vi "old_Ballard - 1553 RT Driver VI.vi"(7 "Operation":T1, 11 "Device Reference in":T2 format="%.0x") -> (0 "Error Code":i32)   [LabVIEW 2017]
uses:
  <vilib>/NI Veristand/Custom Device API/Custom Device Item Ref.ctl
  <vilib>/NI Veristand/Custom Device API/Hardware Interface Driver VI Operation.ctl
  RT Driver/Controls/RT StateVariables.ctl
  <vilib>/NI/NIVS Inline Async API/_VS Inline Async API/VS Inline Async API/VS Inline Async API.lvclass
  RT Driver/Controls/Card Parameters.ctl
  Shared/Controls and Global/Initialization Method.ctl
  <vilib>/NI Veristand/Custom Device API/Data Reference.ctl
  RT Driver/Controls/RT Inline Data_Data Description_Channel.ctl
  RT Driver/Controls/RT Inline Frame Descriptor.ctl
  RT Driver/Controls/RT Inline Frame Descriptor_BC.ctl
  <vilib>/NI Veristand/Custom Device API/Block Data Reference.ctl
  RT Driver/Controls/RT Inline Frame Descriptor_RT.ctl
  Shared/Controls and Global/RT CWD2.ctl
  Shared/Controls and Global/RT CWD1.ctl
  Shared/Controls and Global/RT messageType.ctl
  RT Driver/Controls/Inline_Status_Channels.ctl
  <vilib>/NI Veristand/Custom Device API/Custom Device API.lvlib
  <vilib>/NI VeriStand/Custom Device Tools/Custom Device Utility Library/Custom Device Utility Library.lvlib
  Ballard MIL-1553 Engine.lvlib
  Shared/Ballard 1553 Shared.lvlib
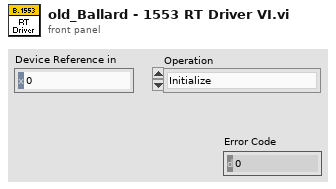
[diagram p1: front panel]
types:
  T1 = typedef "Custom Device API.lvlib/Hardware Interface Driver VI Operation.ctl" = enum16{"Initialize", "Start", "Read Data from HW", "Write Data to HW", "Close"}
  T2 = typedef "Custom Device API.lvlib/Custom Device Item Ref.ctl" = u64
  T3 = typedef "Ballard MIL-1553 Engine.lvlib/RT StateVariables.ctl" = cluster{"Async":refnum<class "VS Inline Async API.lvclass">, "Card Parameters (out)":T4, "Inline Status Channels Refs":T6[], "RT Inline Data_Data Description_Channels":T7[]}
  T4 = typedef "Ballard MIL-1553 Engine.lvlib/Card Parameters.ctl" = cluster{"card number":i32, "core number":i32, "core handle":u64, "core reader handle":u64, "channel handles[]":u64[], "Initialization Method":T5, "PXI slot number":i32}
  T5 = typedef "Ballard 1553 Shared.lvlib/Initialization Method.ctl" = enum16{"PXI Slot Number", "Card Number"}
  T6 = typedef "Custom Device API.lvlib/Data Reference.ctl" = i32
  T7 = typedef "Ballard MIL-1553 Engine.lvlib/RT Inline Data_Data Description_Channel.ctl" = cluster{"hardwareChannel":u16, "First Index for RT2RT Frames":i32, "Frame Drescriptors":T8[]}
  T8 = typedef "Ballard MIL-1553 Engine.lvlib/RT Inline Frame Descriptor.ctl" = cluster{"BC":T9, "RT":T11, "Initialized?":bool, "RT to RT?":bool, "CWD2":T12, "CWD1":T13, "messageType":T14, "Name":string}
  T9 = typedef "Ballard MIL-1553 Engine.lvlib/RT Inline Frame Descriptor_BC.ctl" = cluster{"Timestamp?":bool, "Timestamp Channel Ref":T2, "Data Words?":bool, "Words Block Data Refs":T10[], "Sw1?":bool, "Sw2?":bool, "Status Channel Refs":T2[]}
  T10 = typedef "Custom Device API.lvlib/Block Data Reference.ctl" = cluster{"Data Reference":T6, "Offset":u64, "Length":u64}
  T11 = typedef "Ballard MIL-1553 Engine.lvlib/RT Inline Frame Descriptor_RT.ctl" = cluster{"Timestamp?":bool, "Timestamp Channel Ref":T2, "Data Words?":bool, "Words Block Data Refs":T10[], "Status Channel Ref?":bool, "Status Channel Ref":T2}
  T12 = typedef "Ballard 1553 Shared.lvlib/RT CWD2.ctl" = cluster{"TA (RT)":i8, "SA":i8, "Words (WC)":i8}
  T13 = typedef "Ballard 1553 Shared.lvlib/RT CWD1.ctl" = cluster{"TA (RT)":i8, "SA":i8, "Mode Code":i8, "Words Count":i8}
  T14 = typedef "Ballard 1553 Shared.lvlib/RT messageType.ctl" = enum16{"BC to RT", "RT to BC", "RT to RT", "MC (Rx)", "MC (Tx)"}
  T15 = typedef "Ballard MIL-1553 Engine.lvlib/Inline_Status_Channels.ctl" = enum16{"Error Code", "Inline Read Time (us)", "Inline Write Time (us)", "Unconfigured Frames Counter", "Monitor - Error Counter", "General Protocol Error Counter", "Wrong Sync Error Counter", "Improper Number of Data Words Error", "Manchester Error Counter", "Parity Error Counter", "Word Error Counter"}
  T16 = typedef "Ballard MIL-1553 Engine.lvlib/RT Async Data.ctl" = cluster{"Map (BC to RT)":T17[], "Raw Values (BC to RT)":T19, "Map (RT to ..)":T21[], "Raw Values (RT to ..)":T19, "Map (RTs Status)":T22[], "Raw Values (RTs Status)":T19, "Map (Bc Command Channels)":T23[], "MAP (BC Acyclic Messages Trigger)":T24[], "Map (RT Command Channels)":T25[], "Map (MC Rx)":T26[]}
  T17 = typedef "Ballard MIL-1553 Engine.lvlib/RT Async_Map BC2RT.ctl" = cluster{"Channel Index":i32, "ID":i32, "Channel Data Reference":T6, "Word Index":i32, "Message Handle":u64, "Type":T18}
  T18 = typedef "Ballard MIL-1553 Engine.lvlib/RT Async_Map_Type.ctl" = enum16{"Word (BC to RT)", "Word (MC (Rx))", "Acyclic Message Trigger", "Word (RT to ..)", "Word (RT to RT)", "Word (MC (Tx))", "RT Status", "BC Commands", "RT Commands"}
  T19 = typedef "Ballard MIL-1553 Engine.lvlib/RT Async_Raw Values.ctl" = cluster{"Association":T20[], "Raw Values Array":u16[]}
  T20 = typedef "Ballard MIL-1553 Engine.lvlib/RT Async_Raw Values_Association.ctl" = cluster{"Channel Data Reference":T6, "Raw Value Index":i32}
  T21 = typedef "Ballard MIL-1553 Engine.lvlib/RT Async_Map RT2BC.ctl" = cluster{"Channel Index":i32, "ID":i32, "Word Data Reference":T6, "Word Index":i32, "rt Transfer Handle":u64, "Type":T18}
  T22 = typedef "Ballard MIL-1553 Engine.lvlib/RT Async_Map RTs Status.ctl" = cluster{"Channel Index":i32, "ID":i32, "rt Transfer Handle":u64, "Type":T18}
  T23 = typedef "Ballard MIL-1553 Engine.lvlib/RT Async_Map BC Command Channels.ctl" = cluster{"Channel Index":i32, "ID":i32, "BC Handle":u64, "Type":T18, "BC Command Channel Ref":T2, "Command Type":enum16{"Start Command", "Stop Command"}}
  T24 = typedef "Ballard MIL-1553 Engine.lvlib/RT Async_Map BC Acyclic Messages Trigger.ctl" = cluster{"Channel Index":i32, "BC Handle":u64, "Type":T18, "Acyclic Message Trigger Channel Ref":T2, "Message Name":string}
  T25 = typedef "Ballard MIL-1553 Engine.lvlib/RT Async_Map RT Command Channels.ctl" = cluster{"Channel Index":i32, "ID":i32, "RT Handle":u64, "Type":T18, "RT Command Channel Ref":T2, "Command Type":enum16{"Start Command", "Stop Command"}}
  T26 = typedef "Ballard MIL-1553 Engine.lvlib/RT Async_Map MC Rx.ctl" = cluster{"Channel Index":i32, "ID":i32, "Channel Data Reference":T6, "Word Index":i32, "Message Handle":u64, "Type":T18}
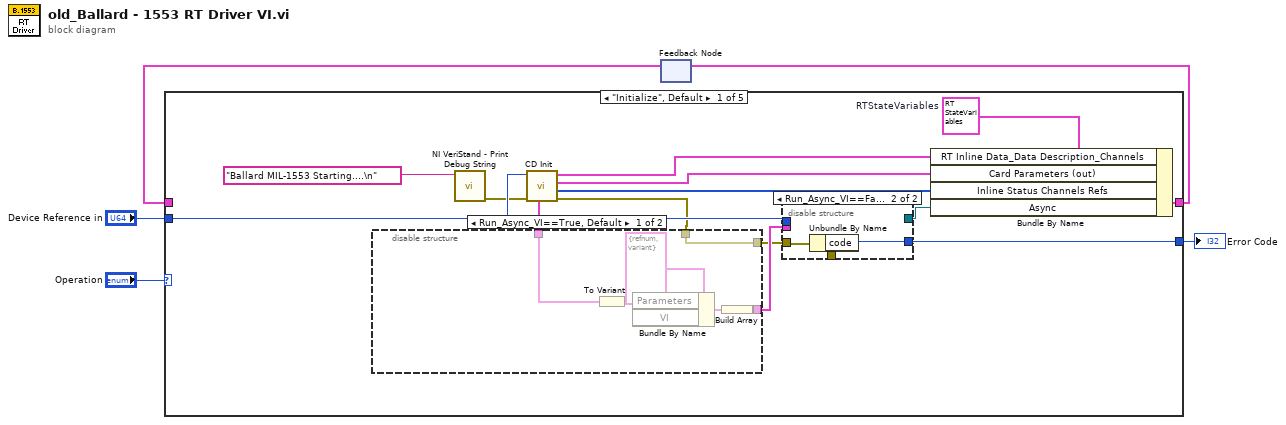
[diagram p0: block diagram]
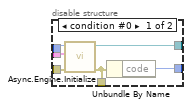
[diagram p3: hidden frame]
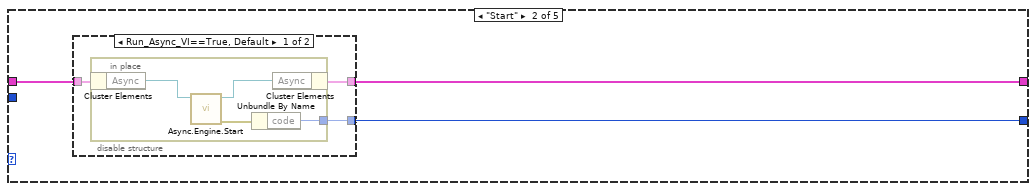
[diagram p4: hidden frame]
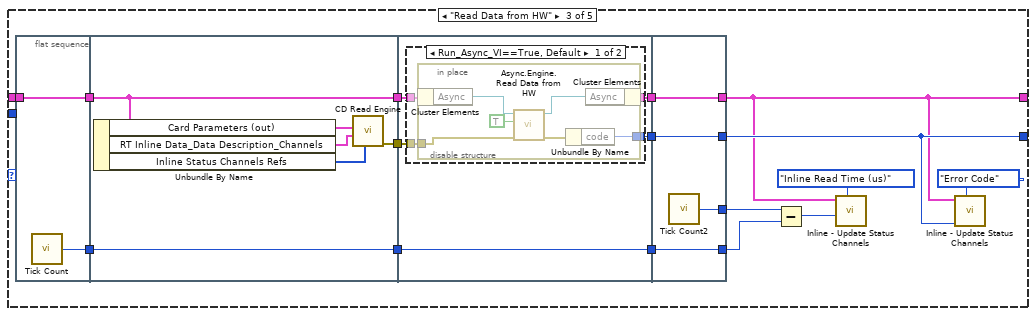
[diagram p6: hidden frame]
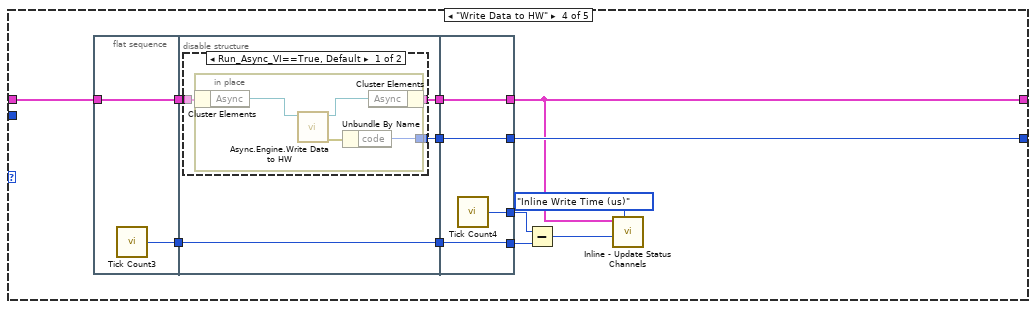
[diagram p8: hidden frame]
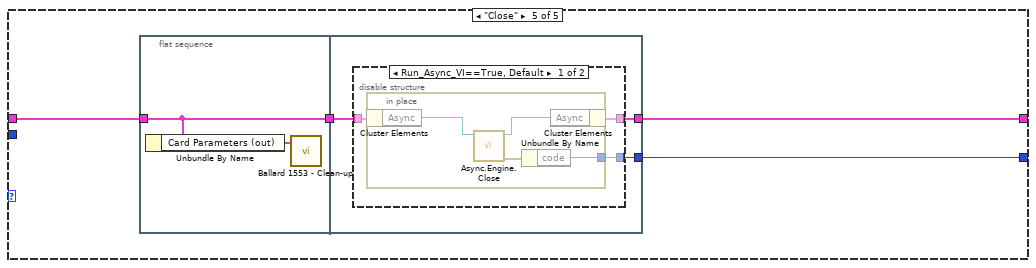
[diagram p10: hidden frame]
diagram:
  n1 = feedback #1() -> (w3:T3)  [unwired: 1 out]
  n2 = case shown="\"Initialize\", Default" "Operation" {
    tunnel: [w17 w36 w53 w91 w122] -> w4
    tunnel: w3 -> [_ w37 w61 w100 w123]
    tunnel: "Device Reference in" -> [w13 _ _ _ _]
    tunnel: [w19 w35 w56 w101 w121] -> w1
    frame "Initialize", Default {
      w16 = T3 {"Async"=refnum, "Card Parameters (out)"={"card number"=0, "core number"=0, "core handle"=0, "core reader handle"=0, "channel handles[]"=[], "Initialization Method"=enum."PXI Slot Number", "PXI slot number"=0}, "Inline Status Channels Refs"=[], "RT Inline Data_Data Description_Channels"=[]}  # RTStateVariables
      n3 = call <vilib>:"NI VeriStand - Print Debug String.vi"("Message"="Ballard MIL-1553 Starting....\n") -> ("error out"=w9:errorcluster)  [unwired: 10 in]
      n4 = call "CD Init.vi"("Error (in)"=w9, "Device Reference"=w13) -> ("Error (out)"=w7:errorcluster, "Inline Status Channels Refs"=w10:T6[], "Card Parameters (out)"=w11:T4, "RT Inline Data_Data Description_Channels"=w12:T7[], "RT Async Data"=w8:T16)  [unwired: 5 in]
      n5 = disable-structure shown="Run_Async_VI==True, Default" {
        disable-tunnel: [w23 _] -> w15
        disable-tunnel: w8 -> [w21 _]
        disable-tunnel: w7 -> [w20 w26]
        disable-tunnel: [w20 w26] -> w6
        frame condition #0 {
          n6 = To Variant(anything=w21) -> (Variant=w22:variant)
          n7 = Bundle By Name(cluster=cluster{"VI":refnum<vi>, "Parameters":variant} {"VI"=refnum, "Parameters"=variant} ("Process"), "Parameters"=w22) -> (w24:cluster{"VI":refnum<vi>, "Parameters":variant})  [unwired: 1 in]
          n8 = Build Array(w24) -> (w23:cluster{"VI":refnum<vi>, "Parameters":variant}[])
        }
        frame condition #1 (active) {
        }
      }
      n9 = disable-structure shown="Run_Async_VI==False" {
        disable-tunnel: [w32 w33] -> w19
        disable-tunnel: [w31 _] -> w18
        disable-tunnel: w15 -> [w30 _]
        disable-tunnel: w6 -> [w29 w34]
        disable-tunnel: w13 -> [w28 _]
        disable-tunnel: [w27 _] -> _
        frame condition #0 {
          n10 = call <vilib>:"Async.Engine.Initialize.vi"("error in (no error)"=w29, "Processes"=w30, "Custom Device Ref"=w28) -> ("error out"=w27:errorcluster, "Async"=w31:refnum<class "VS Inline Async API.lvclass">)  [unwired: 7 in]
          n11 = Unbundle By Name(w27) -> ("code"=w32:i32)
        }
        frame condition #1 (active) {
          n12 = Unbundle By Name(w34) -> ("code"=w33:i32)
        }
      }
      n13 = Bundle By Name(cluster=w16, "RT Inline Data_Data Description_Channels"=w12, "Card Parameters (out)"=w11, "Inline Status Channels Refs"=w10, "Async"=w18) -> (w17:T3)
    }
    frame "Start" {
      n14 = disable-structure shown="Run_Async_VI==True, Default" {
        disable-tunnel: w37 -> [w40 w45]
        disable-tunnel: [w39 w45] -> w36
        disable-tunnel: [w38 _] -> w35
        frame condition #0 {
          n15 = in-place {
            in-place-border: [w41] -> w38
            n16 = in-place-cluster #2(w40) -> ("Async"=w44:refnum<class "VS Inline Async API.lvclass">)
            n17 = call <vilib>:"Async.Engine.Start.vi"("VS Inline Async API in"=w44) -> ("error out"=w42:errorcluster, "VS Inline Async API out"=w43:refnum<class "VS Inline Async API.lvclass">)  [unwired: 9 in]
            n18 = Unbundle By Name(w42) -> ("code"=w41:i32)
            n19 = in-place-cluster #2("Async"=w43) -> (w39:T3)
          }
        }
        frame condition #1 (active) {
        }
      }
    }
    frame "Read Data from HW" {
      n20 = flat-sequence {
        tunnel: w61 -> [w63]
        tunnel: [w63] -> w60
        tunnel: [w62] -> w59
        tunnel: [w68] -> w52
        tunnel: [w69] -> w50
        tunnel: w59 -> [w69]
        tunnel: w60 -> [w68]
        tunnel: [w67] -> w47
        tunnel: w52 -> [w72]
        tunnel: [w71] -> w51
        tunnel: w50 -> [w74]
        tunnel: [w74] -> w49
        tunnel: [w73] -> w48
        tunnel: w47 -> [w70]
        tunnel: [w88] -> w53
        tunnel: [w89] -> w56
        tunnel: w51 -> [w88]
        tunnel: [w87] -> w58
        tunnel: w49 -> [w86]
        tunnel: [w86] -> w57
        tunnel: w48 -> [w89]
        frame #0 {
          n21 = call "Tick Count"() -> ("Tick Count(uSec)"=w62:u32)
        }
        frame #1 {
          n22 = Unbundle By Name(w68) -> ("Card Parameters (out)"=w66:T4, "RT Inline Data_Data Description_Channels"=w64:T7[], "Inline Status Channels Refs"=w65:T6[])
          n23 = call "CD Read Engine.vi"("Inline Status Channels Refs"=w65, "RT Inline Data_Data Description_Channels"=w64, "Card Parameters (in)"=w66) -> ("Error (out)"=w67:errorcluster)  [unwired: 7 in]
        }
        frame #2 {
          n24 = disable-structure shown="Run_Async_VI==True, Default" {
            disable-tunnel: [w78 _] -> w73
            disable-tunnel: w72 -> [w77 w85]
            disable-tunnel: [w76 w85] -> w71
            disable-tunnel: w70 -> [w75 _]
            frame condition #0 {
              n25 = in-place {
                in-place-border: [w82] -> w78
                in-place-border: w75 -> [w79]
                n26 = in-place-cluster #3(w77) -> ("Async"=w84:refnum<class "VS Inline Async API.lvclass">)
                n27 = call <vilib>:"Async.Engine.Read Data from HW.vi"("error in"=w79, "Report Error to Inline?"=TRUE, "Async in"=w84) -> ("error out"=w81:errorcluster, "Async out"=w83:refnum<class "VS Inline Async API.lvclass">)  [unwired: 7 in]
                n28 = Unbundle By Name(w81) -> ("code"=w82:i32)
                n29 = in-place-cluster #3("Async"=w83) -> (w76:T3)
              }
            }
            frame condition #1 (active) {
            }
          }
        }
        frame #3 {
          n30 = call "Tick Count2"() -> ("Tick Count(uSec)"=w87:u32)
        }
      }
      n31 = Subtract(x=w58, y=w57) -> (x-y=w54:u32)
      n32 = call "Inline - Update Status Channels.vi"("Status Channel"=Inline_Status_Channels."Inline Read Time (us)", "Time (us)"=w54, "RTStateVariables"=w53) -> ()  [unwired: 9 in]
      n33 = call "Inline - Update Status Channels.vi"("Status Channel"=Inline_Status_Channels."Error Code", "Error Code"=w56, "RTStateVariables"=w53) -> ()  [unwired: 9 in]
    }
    frame "Write Data to HW" {
      n34 = flat-sequence {
        tunnel: w100 -> [w103]
        tunnel: [w103] -> w99
        tunnel: [w102] -> w96
        tunnel: w99 -> [w104]
        tunnel: [w107] -> w98
        tunnel: [w106] -> w97
        tunnel: w96 -> [w105]
        tunnel: [w105] -> w95
        tunnel: [w118] -> w91
        tunnel: [w119] -> w101
        tunnel: w98 -> [w119]
        tunnel: w97 -> [w118]
        tunnel: [w117] -> w93
        tunnel: w95 -> [w116]
        tunnel: [w116] -> w94
        frame #0 {
          n35 = call "Tick Count3"() -> ("Tick Count(uSec)"=w102:u32)
        }
        frame #1 {
          n36 = disable-structure shown="Run_Async_VI==True, Default" {
            disable-tunnel: [w110 _] -> w107
            disable-tunnel: w104 -> [w109 w115]
            disable-tunnel: [w108 w115] -> w106
            frame condition #0 {
              n37 = in-place {
                in-place-border: [w114] -> w110
                n38 = in-place-cluster #4(w109) -> ("Async"=w112:refnum<class "VS Inline Async API.lvclass">)
                n39 = call <vilib>:"Async.Engine.Write Data to HW.vi"("VS Inline Async API in"=w112) -> ("error out"=w113:errorcluster, "VS Inline Async API out"=w111:refnum<class "VS Inline Async API.lvclass">)  [unwired: 9 in]
                n40 = Unbundle By Name(w113) -> ("code"=w114:i32)
                n41 = in-place-cluster #4("Async"=w111) -> (w108:T3)
              }
            }
            frame condition #1 (active) {
            }
          }
        }
        frame #2 {
          n42 = call "Tick Count4"() -> ("Tick Count(uSec)"=w117:u32)
        }
      }
      n43 = Subtract(x=w93, y=w94) -> (x-y=w92:u32)
      n44 = call "Inline - Update Status Channels.vi"("Status Channel"=Inline_Status_Channels."Inline Write Time (us)", "Time (us)"=w92, "RTStateVariables"=w91) -> ()  [unwired: 9 in]
    }
    frame "Close" {
      n45 = flat-sequence {
        tunnel: w123 -> [w125]
        tunnel: [w125] -> w120
        tunnel: [w127] -> w122
        tunnel: [w126] -> w121
        tunnel: w120 -> [w128]
        frame #0 {
          n46 = Unbundle By Name(w125) -> ("Card Parameters (out)"=w124:T4)
          n47 = call "Ballard 1553 - Clean-up.vi"("Card Parameters"=w124) -> ()  [unwired: 10 in, 1 out]
        }
        frame #1 {
          n48 = disable-structure shown="Run_Async_VI==True, Default" {
            disable-tunnel: w128 -> [w131 w136]
            disable-tunnel: [w130 w136] -> w127
            disable-tunnel: [w129 _] -> w126
            frame condition #0 {
              n49 = in-place {
                in-place-border: [w133] -> w129
                n50 = in-place-cluster #5(w131) -> ("Async"=w135:refnum<class "VS Inline Async API.lvclass">)
                n51 = call <vilib>:"Async.Engine.Close.vi"("Async in"=w135) -> ("error out"=w132:errorcluster, "Async out"=w134:refnum<class "VS Inline Async API.lvclass">)  [unwired: 9 in]
                n52 = Unbundle By Name(w132) -> ("code"=w133:i32)
                n53 = in-place-cluster #5("Async"=w134) -> (w130:T3)
              }
            }
            frame condition #1 (active) {
            }
          }
        }
      }
    }
  }
  "Error Code" <- w1
  n54 = feedback-in #1(w4) -> ()
